vi "Calcuate Flow Parameters.vi"(8 "error in (no error)":errorcluster, 10 "Hardware Configuration":T2={"Head type"=enum."High Flow", "Pressure range"=enum."High pressure", "Stator material"=enum."PTFE", "Rotor material"=enum."Ceramic", "Rotor O-ring material"=enum."none", "Piston O-ring material"=enum."Viton", "Pump body material"=enum."Stainless steel", "Controller"=enum."MForce", "Gear ratio"=enum."9.87", "Motor resolution"=enum."1.8", "Equipped with encoder"=enum."No"}, 11 "VISA resource in":refnum<visa-resource-name>) -> (0 "error out":errorcluster, 2 "Flow Configuration":T1, 3 "VISA resource out":refnum<visa-resource-name>)   [LabVIEW 2020, in "Global FIA milliGAT.lvlib"]
uses:
  <instrlib>/RxnRover/Global FIA milliGAT 3.14/Global FIA milliGAT.lvlib
  <instrlib>/RxnRover/Global FIA milliGAT 3.14/Public/Utility/Low Level/Hardware Configuration.ctl
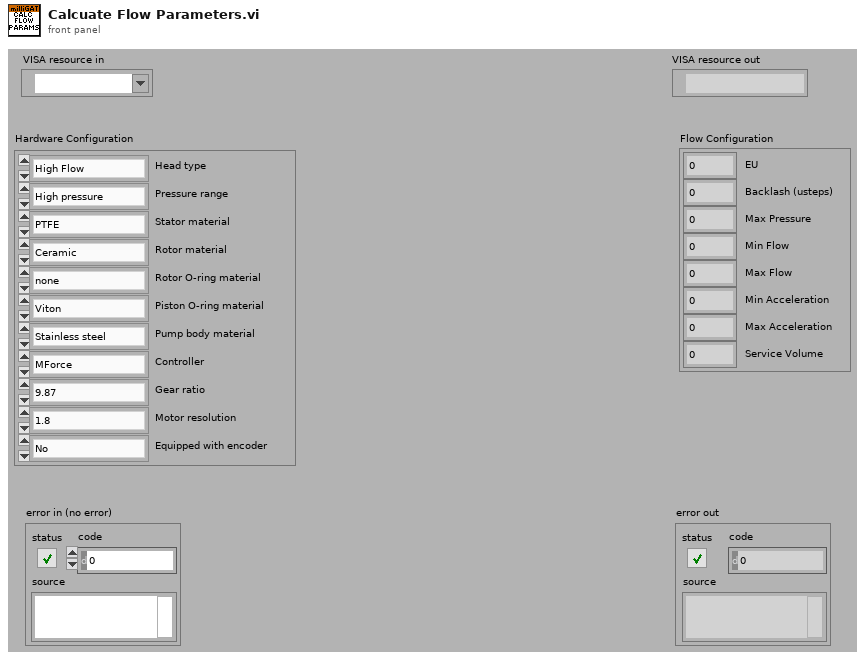
[diagram p1: front panel]
types:
  T1 = cluster{"EU":dbl, "Backlash (usteps)":dbl, "Max Pressure":dbl, "Min Flow":dbl, "Max Flow":dbl, "Min Acceleration":dbl, "Max Acceleration":dbl, "Service Volume":dbl}
  T2 = typedef "Global FIA milliGAT.lvlib/Hardware Configuration.ctl" = cluster{"Head type":enum16{"Low Flow", "High Flow"}, "Pressure range":enum16{"Low pressure", "High pressure"}, "Stator material":enum16{"PTFE", "Valcon E3", "PEEK/PTFE", "Valcon H2"}, "Rotor material":enum16{"Ceramic", "Valcon P", "CTFE"}, "Rotor O-ring material":enum16{"none", "Viton", "Kalrez"}, "Piston O-ring material":enum16{"Viton", "Kalrez"}, "Pump body material":enum16{"Stainless steel", "Aluminum"}, "Controller":enum16{"MForce", "MDrive"}, "Gear ratio":enum16{"4.75", "9.87", "15", "22.56"}, "Motor resolution":enum16{"1.8", "0.9"}, "Equipped with encoder":enum16{"No", "Yes"}}
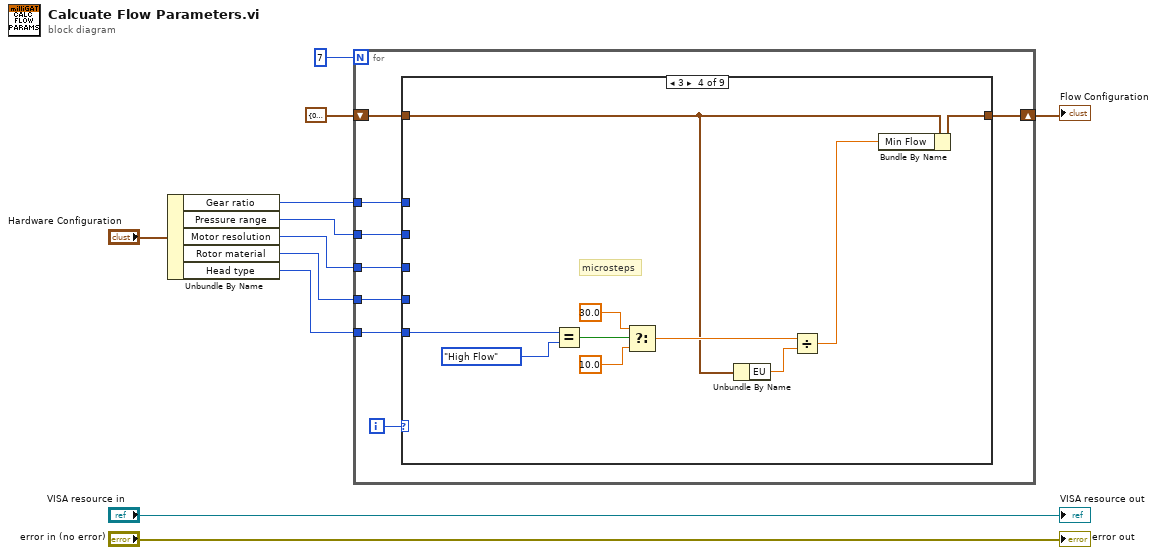
[diagram p0: block diagram]
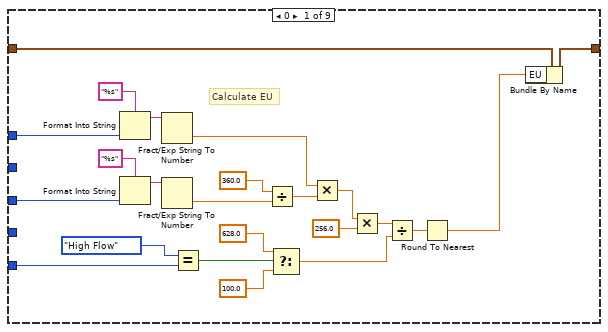
[diagram p2: hidden frame]
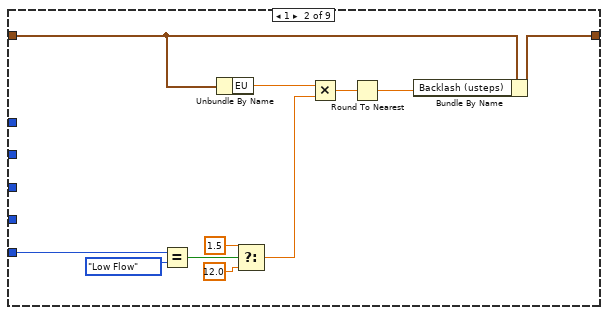
[diagram p3: hidden frame]
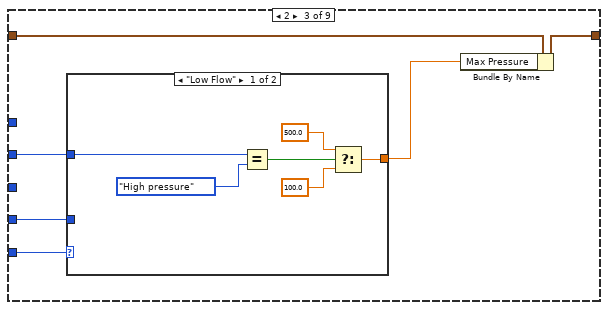
[diagram p4: hidden frame]
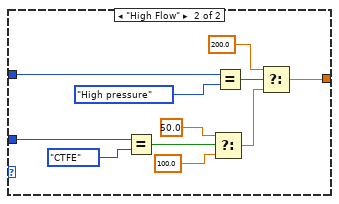
[diagram p5: hidden frame]
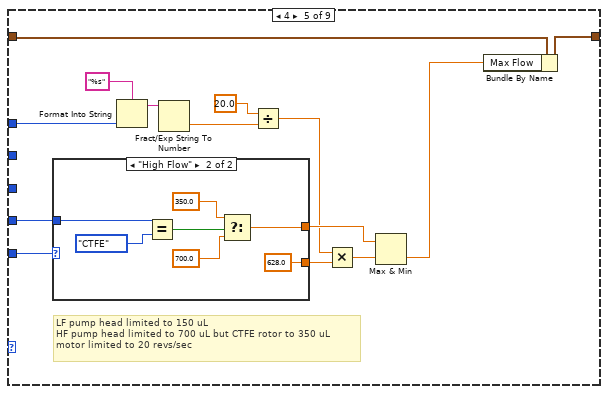
[diagram p6: hidden frame]
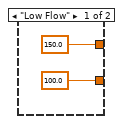
[diagram p7: hidden frame]
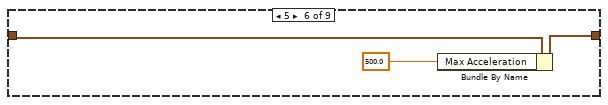
[diagram p8: hidden frame]
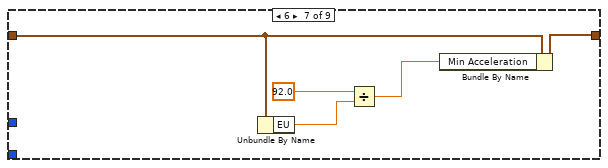
[diagram p9: hidden frame]
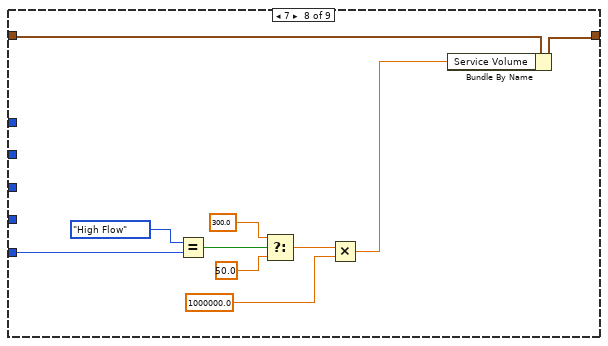
[diagram p10: hidden frame]
diagram:
  n1 = Unbundle By Name("Hardware Configuration") -> ("Gear ratio"=w9:enum16{"4.75", "9.87", "15", "22.56"}, "Pressure range"=w8:enum16{"Low pressure", "High pressure"}, "Motor resolution"=w7:enum16{"1.8", "0.9"}, "Rotor material"=w6:enum16{"Ceramic", "Valcon P", "CTFE"}, "Head type"=w5:enum16{"Low Flow", "High Flow"})
  n2 = for {
    N: 7 -> [_]
    tunnel: w5 -> [w18]
    tunnel: w6 -> [w17]
    tunnel: w9 -> [w16]
    tunnel: w7 -> [w15]
    tunnel: w8 -> [w14]
    shift-right: [w13] -> w4
    shift-left: T1 {"EU"=0.0, "Backlash (usteps)"=0.0, "Max Pressure"=0.0, "Min Flow"=0.0, "Max Flow"=0.0, "Min Acceleration"=0.0, "Max Acceleration"=0.0, "Service Volume"=0.0} ("Flow Configuration") -> [w12]
    i -> [w19]
    n3 = case shown="3" w19 {
      tunnel: w18 -> [w42 w43 w59 w81 w93 _ _ w121 _]
      tunnel: w17 -> [_ _ w58 _ w92 _ _ _ _]
      tunnel: w16 -> [w41 _ _ _ w91 _ _ _ _]
      tunnel: w15 -> [w40 _ _ _ _ _ _ _ _]
      tunnel: w14 -> [_ _ w57 _ _ _ _ _ _]
      tunnel: [w39 w44 w56 w80 w89 w112 w116 w120 w128] -> w13
      tunnel: w12 -> [w38 w45 w55 w78 w88 w111 w114 w119 w128]
      frame 0 {
        # "Calculate EU"
        n4 = Format Into String(format string="%s", w41) -> (resulting string=w30:string)  [unwired: 2 in, 1 out]
        n5 = Format Into String(format string="%s", w40) -> (resulting string=w25:string)  [unwired: 2 in, 1 out]
        n6 = Fract/Exp String To Number(string=w30) -> (number=w28:dbl)  [unwired: 3 in, 1 out]
        n7 = Fract/Exp String To Number(string=w25) -> (number=w24:dbl)  [unwired: 3 in, 1 out]
        n8 = Equal?(x=enum16{"Low Flow", "High Flow"}."High Flow", y=w42) -> (x = y?=w35:bool)
        n9 = Divide(x=360.0, y=w24) -> (x/y=w29:dbl)
        n10 = Select(t=628.0, s=w35, f=100.0) -> (s? t:f=w27:dbl)
        n11 = Multiply(x=w28, y=w29) -> (x*y=w22:dbl)
        n12 = Multiply(x=w22, y=256.0) -> (x*y=w20:dbl)
        n13 = Divide(x=w20, y=w27) -> (x/y=w23:dbl)
        n14 = Round To Nearest(number=w23) -> (nearest integer value=w37:dbl)
        n15 = Bundle By Name(cluster=w38, "EU"=w37) -> (w39:T1)
      }
      frame 1 {
        n16 = Equal?(x=w43, y=enum16{"Low Flow", "High Flow"}."Low Flow") -> (x = y?=w52:bool)
        n17 = Unbundle By Name(w45) -> ("EU"=w49:dbl)
        n18 = Select(t=1.5, s=w52, f=12.0) -> (s? t:f=w48:dbl)
        n19 = Multiply(x=w49, y=w48) -> (x*y=w47:dbl)
        n20 = Round To Nearest(number=w47) -> (nearest integer value=w46:dbl)
        n21 = Bundle By Name(cluster=w45, "Backlash (usteps)"=w46) -> (w44:T1)
      }
      frame 2 {
        n22 = case shown="\"Low Flow\"" w59 {
          tunnel: w57 -> [w65 w76]
          tunnel: [w62 w72] -> w54
          tunnel: w58 -> [_ w71]
          frame "Low Flow" {
            n23 = Equal?(x=w65, y=enum16{"Low pressure", "High pressure"}."High pressure") -> (x = y?=w63:bool)
            n24 = Select(t=500.0, s=w63, f=100.0) -> (s? t:f=w62:dbl)
          }
          frame "High Flow" {
            n25 = Equal?(x=w71, y=enum16{"Ceramic", "Valcon P", "CTFE"}."CTFE") -> (x = y?=w68:bool)
            n26 = Select(t=50.0, s=w68, f=100.0) -> (s? t:f=w66:dbl)
            n27 = Equal?(x=w76, y=enum16{"Low pressure", "High pressure"}."High pressure") -> (x = y?=w74:bool)
            n28 = Select(t=200.0, s=w74, f=w66) -> (s? t:f=w72:dbl)
          }
        }
        n29 = Bundle By Name(cluster=w55, "Max Pressure"=w54) -> (w56:T1)
      }
      frame 3 {
        # "microsteps"
        n30 = Equal?(x=w81, y=enum16{"Low Flow", "High Flow"}."High Flow") -> (x = y?=w85:bool)
        n31 = Select(t=30.0, s=w85, f=10.0) -> (s? t:f=w82:dbl)
        n32 = Unbundle By Name(w78) -> ("EU"=w77:dbl)
        n33 = Divide(x=w82, y=w77) -> (x/y=w79:dbl)
        n34 = Bundle By Name(cluster=w78, "Min Flow"=w79) -> (w80:T1)
      }
      frame 4 {
        # "LF pump head limited to 150 uL\nHF pump head limited to 700 uL but CTFE rotor to 350 uL \nmotor limited to 20 revs/sec"
        n35 = case shown="\"High Flow\"" w93 {
          tunnel: w92 -> [_ w109]
          tunnel: [150.0 ("f") w104] -> w98
          tunnel: [100.0 628.0] -> w95
          frame "Low Flow" {
          }
          frame "High Flow" {
            n36 = Equal?(x=w109, y=enum16{"Ceramic", "Valcon P", "CTFE"}."CTFE") -> (x = y?=w107:bool)
            n37 = Select(t=350.0, s=w107, f=700.0) -> (s? t:f=w104:dbl)
          }
        }
        n38 = Format Into String(format string="%s", w91) -> (resulting string=w99:string)  [unwired: 2 in, 1 out]
        n39 = Fract/Exp String To Number(string=w99) -> (number=w96:dbl)  [unwired: 3 in, 1 out]
        n40 = Divide(x=20.0 ("y"), y=w96) -> (x/y=w90:dbl)
        n41 = Multiply(x=w90, y=w95) -> (x*y=w94:dbl)
        n42 = Max & Min(x=w98, y=w94) -> (min(x,y)=w87:dbl)  [unwired: 1 out]
        n43 = Bundle By Name(cluster=w88, "Max Flow"=w87) -> (w89:T1)
      }
      frame 5 {
        n44 = Bundle By Name(cluster=w111, "Max Acceleration"=500.0 ("f")) -> (w112:T1)
      }
      frame 6 {
        n45 = Unbundle By Name(w114) -> ("EU"=w113:dbl)
        n46 = Divide(x=92.0 ("f"), y=w113) -> (x/y=w115:dbl)
        n47 = Bundle By Name(cluster=w114, "Min Acceleration"=w115) -> (w116:T1)
      }
      frame 7 {
        n48 = Equal?(x=enum16{"Low Flow", "High Flow"}."High Flow" ("y"), y=w121) -> (x = y?=w126:bool)
        n49 = Select(t=300.0, s=w126, f=50.0) -> (s? t:f=w123:dbl)
        n50 = Multiply(x=w123, y=1000000.0) -> (x*y=w118:dbl)
        n51 = Bundle By Name(cluster=w119, "Service Volume"=w118) -> (w120:T1)
      }
      frame Default {
      }
    }
  }
  "Flow Configuration" <- w4
  "VISA resource out" <- "VISA resource in"
  "error out" <- "error in (no error)"
